vi "String.Append to Log_V2.vi"(6 "Add Time":bool, 7 "MaxLen":i32=10000, 8 "Delimiter":string="\t", 9 "Prefix":string, 10 "New Data":string, 11 "Data":string) -> (3 "Data Out":string)   [LabVIEW 2024]
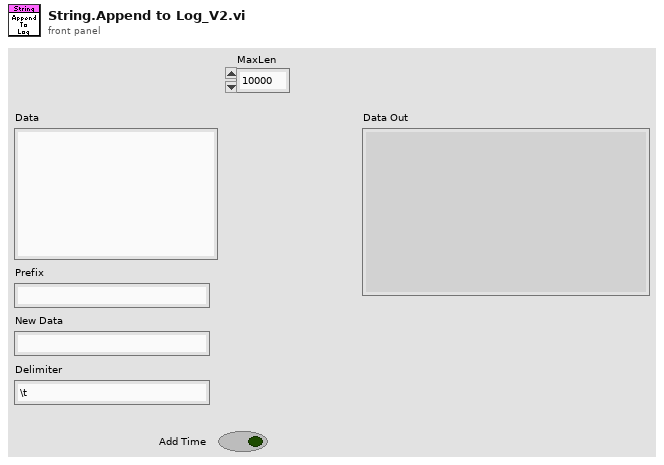
[diagram p1: front panel]
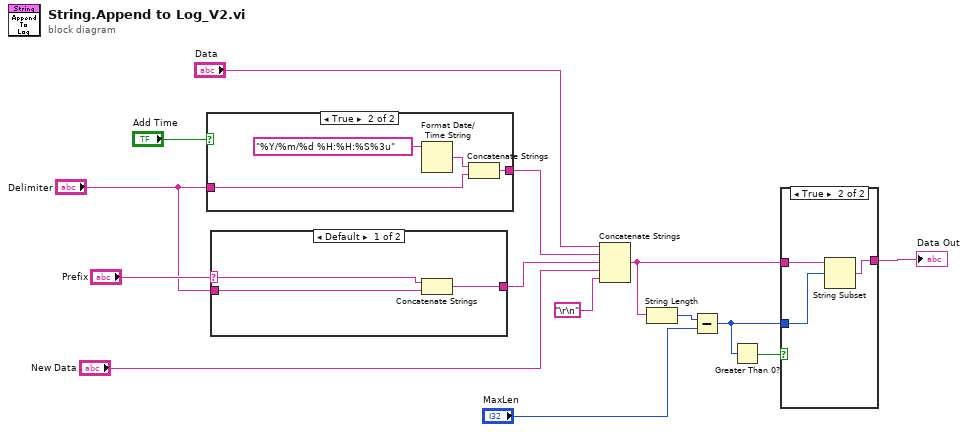
[diagram p0: block diagram]
diagram:
  n1 = case shown="True" "Add Time" {
    tunnel: "Delimiter" -> [_ w16]
    tunnel: [_ w15] -> w10
    frame False {
    }
    frame True {
      n2 = Format Date/Time String(time format string (%c)="%Y/%m/%d %H:%H:%S%3u") -> (date/time string=w17:string)  [unwired: 2 in]
      n3 = Concatenate Strings(w17, w16) -> (w15:string)
    }
  }
  n4 = case shown="Default" "Prefix" {
    selector: "Prefix" -> [w21 _]
    tunnel: "Delimiter" -> [w20 _]
    tunnel: [w19 _] -> w9
    frame Default {
      n5 = Concatenate Strings(w21, w20) -> (w19:string)
    }
    frame "" {
    }
  }
  n6 = Concatenate Strings("Data", w10, w9, "New Data", "\r\n") -> (w2:string)
  n7 = String Length(string=w2) -> (length=w6:i32)
  n8 = Subtract(x=w6, y="MaxLen") -> (x-y=w3:i32)
  n9 = Greater Than 0?(x=w3) -> (x > 0?=w4:bool)
  n10 = case shown="True" w4 {
    tunnel: w3 -> [_ w24]
    tunnel: w2 -> [w22 w25]
    tunnel: [w22 w23] -> w1
    frame False {
    }
    frame True {
      n11 = String Subset(string=w25, offset (0)=w24) -> (substring=w23:string)  [unwired: 1 in]
    }
  }
  "Data Out" <- w1
